vi "Set XY Graph Value Single.vi"(9 "XY Graph Data":T1 {"Y" format="%#_f"; "X" format="%#_f"}, 11 "XY Graph Reference In":refnum<vi>) -> ()   [LabVIEW 2019]
uses:
  TypeDef/XY Graph Data.ctl
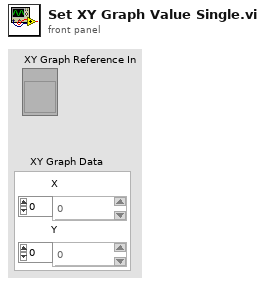
[diagram p1: front panel]
types:
  T1 = typedef "XY Graph Data.ctl" = cluster{"X":dbl[], "Y":dbl[]}
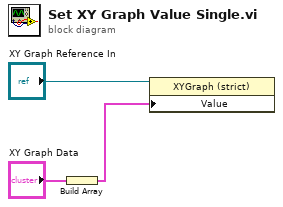
[diagram p0: block diagram]
diagram:
  n1 = Build Array("XY Graph Data") -> (w1:T1[])
  n2 = property class="XYGraph (strict)"(reference="XY Graph Reference In", "Value"=w1) -> ()  [unwired: 1 in, 2 out]
